vi "Close FPGA.vi"(8 "error in (no error)":errorcluster, 11 "Refnum in":refnum<k20>) -> (0 "error out":errorcluster)   [LabVIEW 2016]
uses:
  Typedefs/IO Buffer Operation.ctl
  <vilib>/FPGAPlugInAG/Dynamic/niLvFpga_Close_Dynamic.vi
  <vilib>/rvi/interface/nirviCloseFPGA/nirviCloseFPGA.xnode
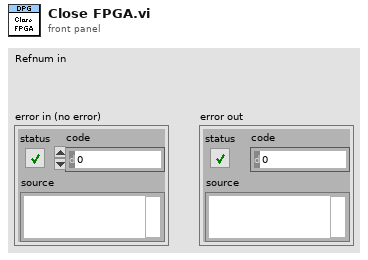
[diagram p1: front panel]
types:
  T1 = typedef "IO Buffer Operation.ctl" = enum16{"Initialize", "Write IO Data_Rd", "Read IO Data_Rd", "Write IO Data_Wr", "Read IO Data_Wr", "Write  IO Data_Dir", "Read  IO Data_Dir", "Write Host to Target FIFO", "Read Host to Target FIFO", "Write Target to Host FIFO", "Read Target to Host FIFO", "Write Monitor Enable?", "Read Monitor Enable?", "Close"}
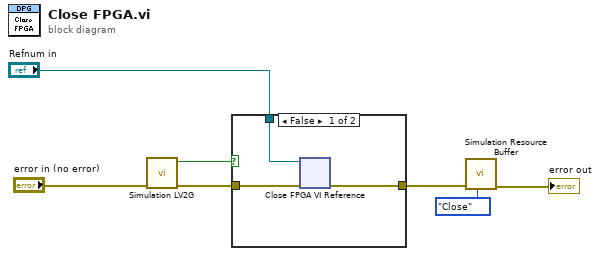
[diagram p0: block diagram]
diagram:
  n1 = call "Simulation LV2G.vi"("error in (no error)"="error in (no error)") -> ("error out"=w5:errorcluster, "Simulation? out"=w4:bool)  [unwired: 9 in]
  n2 = case shown="False" w4 {
    tunnel: [w10 w11] -> w2
    tunnel: "Refnum in" -> [w9 _]
    tunnel: w5 -> [w8 w11]
    frame False {
      n3 = xnode "Close FPGA VI Reference"("FPGA VI Reference In"=w9, "error in"=w8) -> ("error out"=w10:errorcluster)
    }
    frame True {
    }
  }
  n4 = call "Simulation Resource Buffer.vi"("IO Buffer Operation"=IO_Buffer_Operation."Close", "error in (no error)"=w2) -> ("error out"=→"error out":errorcluster)  [unwired: 7 in, 2 out]
